vi "Step from Type.vi"(11 "Step Type":T1) -> (3 "Step":refnum<class "Recipe Step.lvclass">)   [LabVIEW 2018, in "Temp Recipe.lvlib" / "Recipe Editor.lvclass"]
uses:
  Recipe Editor.lvclass
  Step Type.ctl
  Recipe Step/Recipe Step.lvclass
  Target Step/Target Step.lvclass
  C:/dev/source/Systems/NI Week/Temperature Recipe/Temp Recipe/Recipe Step/Recipe Step.lvclass
  Rate Step/Rate Step.lvclass
  Time Step/Time Step.lvclass
  Rate Duration/Rate Duration.lvclass
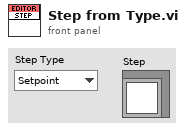
[diagram p1: front panel]
types:
  T1 = typedef "Temp Recipe.lvlib/Recipe Editor.lvclass/Step Type.ctl" = enum16{"Setpoint", "Step Rate", "Rate Duration", "Delay"}
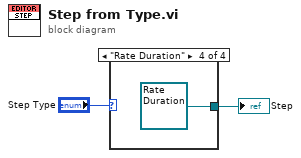
[diagram p0: block diagram]
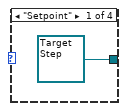
[diagram p2: hidden frame]
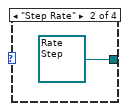
[diagram p3: hidden frame]
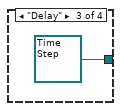
[diagram p4: hidden frame]
diagram:
  n1 = case shown="\"Rate Duration\"" "Step Type" {
    tunnel: [refnum<class "Target Step.lvclass"> refnum ("Temp Recipe.lvlib:Target Step.lvclass") refnum<class "Rate Step.lvclass"> refnum ("Temp Recipe.lvlib:Rate Step.lvclass") refnum<class "Time Step.lvclass"> refnum ("Temp Recipe.lvlib:Time Step.lvclass") refnum<class "Rate Duration.lvclass"> refnum ("Temp Recipe.lvlib:Rate Duration.lvclass")] -> w1
    frame "Setpoint" {
    }
    frame "Step Rate" {
    }
    frame "Delay" {
    }
    frame "Rate Duration" {
    }
  }
  "Step" <- w1
